vi "Get_Latest_NewFI - no check.vi"(11 "Error In":errorcluster) -> (4 "Output Path":path, 15 "Error Out 2":errorcluster)   [LabVIEW 2016]
uses:
  <vilib>/regexp/Match Regular Expression.xnode
  <vilib>/httpClient/LabVIEWHTTPClient.lvlib
  <vilib>/zip/NI_Unzip.lvlib
panel:
  out "Status":string
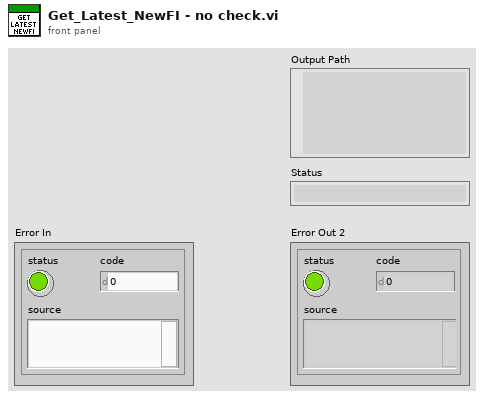
[diagram p1: front panel]
types:
  T1 = typedef "LabVIEWHTTPClient.lvlib/ClientHandle.ctl" = refnum<k1>
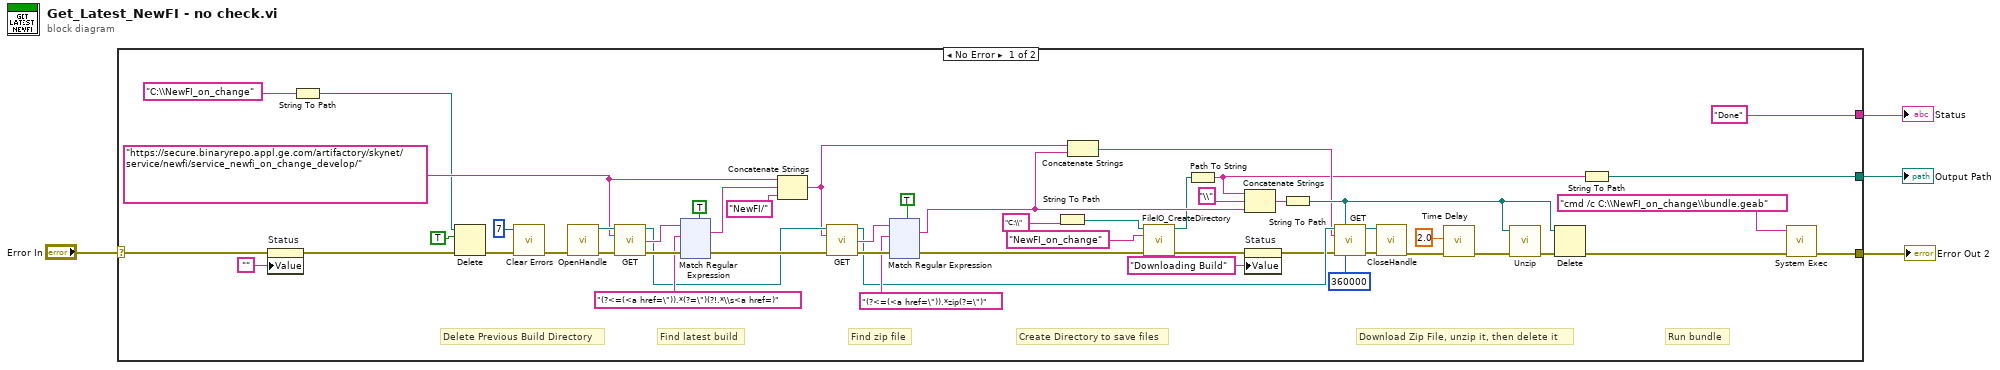
[diagram p0: block diagram]
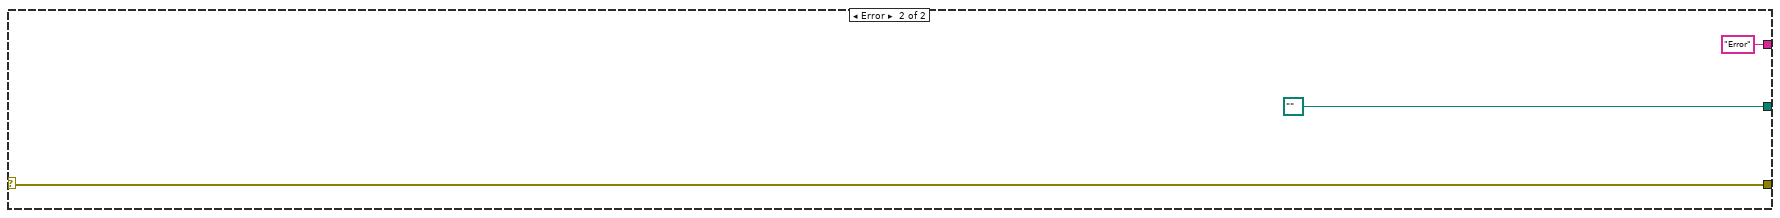
[diagram p2: hidden frame]
diagram:
  n1 = case shown="No Error" "Error In" {
    selector: "Error In" -> [w12 w287]
    tunnel: [w16 w287] -> w2
    tunnel: [w5 path ""] -> w3
    tunnel: ["Done" "Error"] -> w1
    frame No Error {
      w29 = "https://secure.binaryrepo.appl.ge.com/artifactory/skynet/service/newfi/service_newfi_on_change_develop/"
      # "Run bundle"
      # "Delete Previous Build Directory"
      # "Create Directory to save files"
      # "Find zip file"
      # "Find latest build"
      # "Download Zip File, unzip it, then delete it"
      n2 = property on="Status" class="Str"(error in=w12, "Value"="") -> (error out=w11:errorcluster)  [unwired: 1 in, 1 out]
      n3 = String To Path(string="C:\\NewFI_on_change") -> (path=w22:path)
      n4 = Delete(path (use dialog)=w22, entire hierarchy (F)=TRUE, error in=w11) -> (error out=w26:errorcluster)  [unwired: 2 in, 2 out]
      n5 = call <vilib>:"Clear Errors.vi"("error in (no error)"=w26, "specific error code to clear (0: all)"=7) -> ("error out"=w25:errorcluster)  [unwired: 4 in, 1 out]
      n6 = call <vilib>:"OpenHandle.vi"("error in (no error)"=w25) -> ("client handle out"=w55:T1, "error out"=w56:errorcluster)  [unwired: 13 in]
      n7 = call <vilib>:"GET.vi"("client handle"=w55, "url"=w29, "error in (no error)"=w56) -> ("client handle out"=w48:T1, "body"=w53:string, "error out"=w54:errorcluster)  [unwired: 9 in, 1 out]
      n8 = xnode "Match Regular Expression"("input string"=w53, "regular expression"="(?<=(<a href=\")).*(?=\")(?!.*\\s<a href=)", "error in"=w54, "multiline? (F)"=TRUE) -> ("whole match"=w52:string, "error out"=w49:errorcluster)  [unwired: 2 in, 3 out]
      n9 = Concatenate Strings(w29, w52, "NewFI/" ("string")) -> (w35:string)
      n10 = call <vilib>:"GET.vi"("client handle"=w48, "url"=w35, "error in (no error)"=w49) -> ("client handle out"=w41:T1, "body"=w45:string, "error out"=w46:errorcluster)  [unwired: 9 in, 1 out]
      n11 = xnode "Match Regular Expression"("input string"=w45, "regular expression"="(?<=(<a href=\")).*zip(?=\")", "error in"=w46, "multiline? (F)"=TRUE) -> ("whole match"=w34:string, "error out"=w23:errorcluster)  [unwired: 2 in, 3 out]
      n12 = String To Path(string="C:\\") -> (path=w18:path)
      n13 = Concatenate Strings(w35, w34) -> (w33:string)
      n14 = call "FileIO_CreateDirectory.vi"("Base Path"=w18, "Directory Name"="NewFI_on_change", "Error In"=w23) -> ("File Path Control"=w21:path, "Error Out"=w9:errorcluster)  [unwired: 11 in]
      n15 = Path To String(path=w21) -> (string=w15:string)
      n16 = Concatenate Strings(w15, "\\" ("string"), w34) -> (w39:string)
      n17 = property on="Status" class="Str"(error in=w9, "Value"="Downloading Build" ("Status")) -> (error out=w8:errorcluster)  [unwired: 1 in, 1 out]
      n18 = String To Path(string=w39) -> (path=w38:path)
      n19 = call <vilib>:"GET.vi"("client handle"=w41, "output file"=w38, "url"=w33, "error in (no error)"=w8, "timeout (10000)"=360000) -> ("client handle out"=w43:T1, "error out"=w42:errorcluster)  [unwired: 7 in, 2 out]
      n20 = call <vilib>:"CloseHandle.vi"("client handle"=w43, "error in (no error)"=w42) -> ("error out"=w31:errorcluster)  [unwired: 13 in]
      n21 = call "Time Delay"("error in (no error)"=w31, "Delay Time (s)"=2.0) -> ("error out"=w30:errorcluster)  [unwired: 9 in]
      n22 = call <vilib>:"Unzip.vi"("error in (no error)"=w30, "Zip file"=w38) -> ("error out"=w37:errorcluster)  [unwired: 7 in, 2 out]
      n23 = Delete(path (use dialog)=w38, error in=w37) -> (error out=w17:errorcluster)  [unwired: 3 in, 2 out]
      n24 = String To Path(string=w15) -> (path=w5:path)
      n25 = call <vilib>:"System Exec.vi"("error in (no error)"=w17, "command line"="cmd /c C:\\NewFI_on_change\\bundle.geab" ("string")) -> ("error out"=w16:errorcluster)  [unwired: 6 in, 3 out]
    }
    frame Error {
    }
  }
  "Output Path" <- w3
  "Error Out 2" <- w2
  "Status" <- w1
